vi "Routing Channel Page.vi"(8 "error in (no error)":errorcluster, 11 "Node Ptr":T6 format="%.0x") -> (0 "error out":errorcluster)   [LabVIEW 2020, in "Routing and Faulting System Explorer.lvlib"]
uses:
  Routing and Faulting System Explorer.lvlib
  <vilib>/NI VeriStand/Custom Device API/Custom Device Item Ref.ctl
  State-Value Row.ctl
  Connection Row.ctl
  State Control.ctl
  Shared/UI Common/Add Button.ctl
  Routing Channel Page Controls.ctl
  2402a215-ce2b-4427-ab28-3f6d8102afb6.vi
  Shared/Constants.vi
  Shared/UI Common/Set Control Value.vi
  <vilib>/NI VeriStand/Custom Device API/Custom Device API.lvlib
  Scripting/Routing and Faulting Scripting.lvlib
  Shared/UI Common/UI Common.lvlib
  Shared/Routing and Faulting Shared.lvlib
panel:
  in  "Configuration Tab":T1(tab)
  in  "Connections":T2[](array[typedef])
  in  "State Value":string
  in  "State Description":string
  in  "Add Connection":T3
  in  "State Name":T4
  in  "Duplicate State":bool
  in  "Remove State":bool
  in  "Add State":bool
  in  "Previous State":bool
  in  "Next State":bool
  in  "States":T5[](array[typedef])
  in  "Initial State":string(combo)
  in  "Routing Channel Name":string
  in  "SHDocVw.IWebBrowser":refnum<k7>(container)
  in  "Description":string
  # "Source"
  # "Destination"
  # "State Name"
  # "State Value"
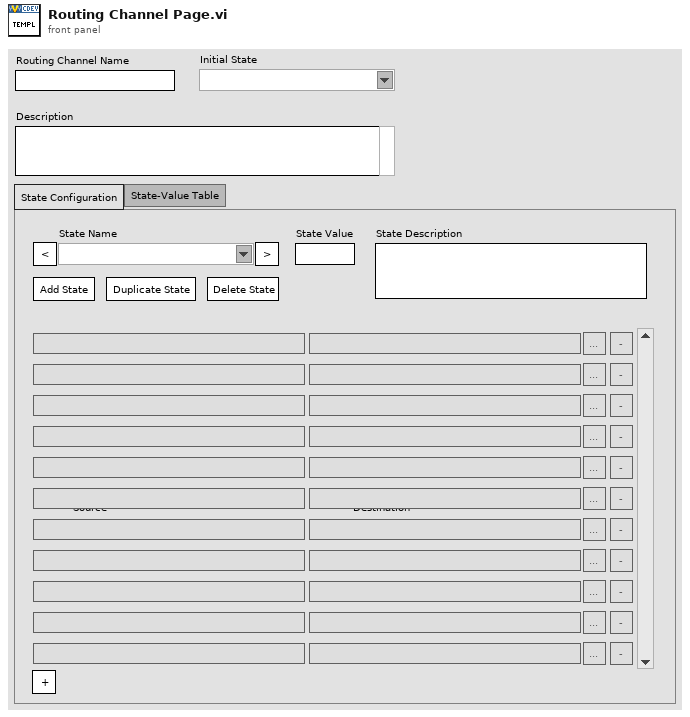
[diagram p1: front panel]
types:
  T1 = enum32{"State Configuration", "State-Value Table"}
  T2 = typedef "Routing and Faulting System Explorer.lvlib/Connection Row.ctl" = cluster{"Source":string, "Destination":string, "Edit":bool, "Remove":bool}
  T3 = typedef "UI Common.lvlib/Add Button.ctl" = bool
  T4 = typedef "Routing and Faulting System Explorer.lvlib/State Control.ctl" = string
  T5 = typedef "Routing and Faulting System Explorer.lvlib/State-Value Row.ctl" = cluster{"State":string, "State Value":string}
  T6 = typedef "Custom Device API.lvlib/Custom Device Item Ref.ctl" = u64
  T7 = typedef "Routing and Faulting System Explorer.lvlib/Routing Channel Page Controls.ctl" = cluster{"Description":refnum<vi>, "Routing Channel Name":refnum<vi>, "Initial State":refnum<vi>, "Configuration Tab":refnum<vi>, "States":refnum<vi>, "State Value":refnum<vi>, "State Name":refnum<vi>, "State Description":refnum<vi>, "Connections":refnum<vi>}
  T8 = typedef "Routing and Faulting Scripting.lvlib/Module Information.ctl" = cluster{"Module Path":string, "Product Name":string, "Possible Connections":T9[], "Configuration Revision":u32, "Validated":bool, "Missing":bool}
  T9 = typedef "Routing and Faulting Hardware API.lvlib/Possible Connections for Endpoint.ctl" = cluster{"Source":string, "Destinations":string[]}
  T10 = typedef "Routing and Faulting System Explorer.lvlib/Channel Editor State.ctl" = cluster{"Modules and Connections":T11[], "Alias Mappings UI":T12[], "Mappings by Module UI":T14[]}
  T11 = typedef "Routing and Faulting System Explorer.lvlib/Possible Connections.ctl" = cluster{" Module Path":string, "Short Module Path":string, "Product Name":string, "Possible Connections":T9[], "Missing":bool}
  T12 = typedef "Routing and Faulting Shared.lvlib/Alias Mapping.ctl" = cluster{"Alias":string, "Endpoint":T13}
  T13 = typedef "Routing and Faulting Shared.lvlib/Alias Endpoint.ctl" = cluster{"Module Path":string, "Endpoint":string}
  T14 = typedef "Routing and Faulting System Explorer.lvlib/Alias Map by Module.ctl" = cluster{"Module":string, "Alias Map":cluster{"Aliases":string[], "Endpoints":string[]}}
  T15 = typedef "Custom Device API.lvlib/Custom Device Commands.ctl" = enum16{"Default", "Item renamed", "Shutdown", "Dynamic button pressed"}
  T16 = typedef "Routing and Faulting Shared.lvlib/Connection.ctl" = cluster{"Module":string, "Source":string, "Destination":string}
  T17 = typedef "LVPoint32TypeDef.ctl" = cluster{"Horizontal":i32, "Vertical":i32}
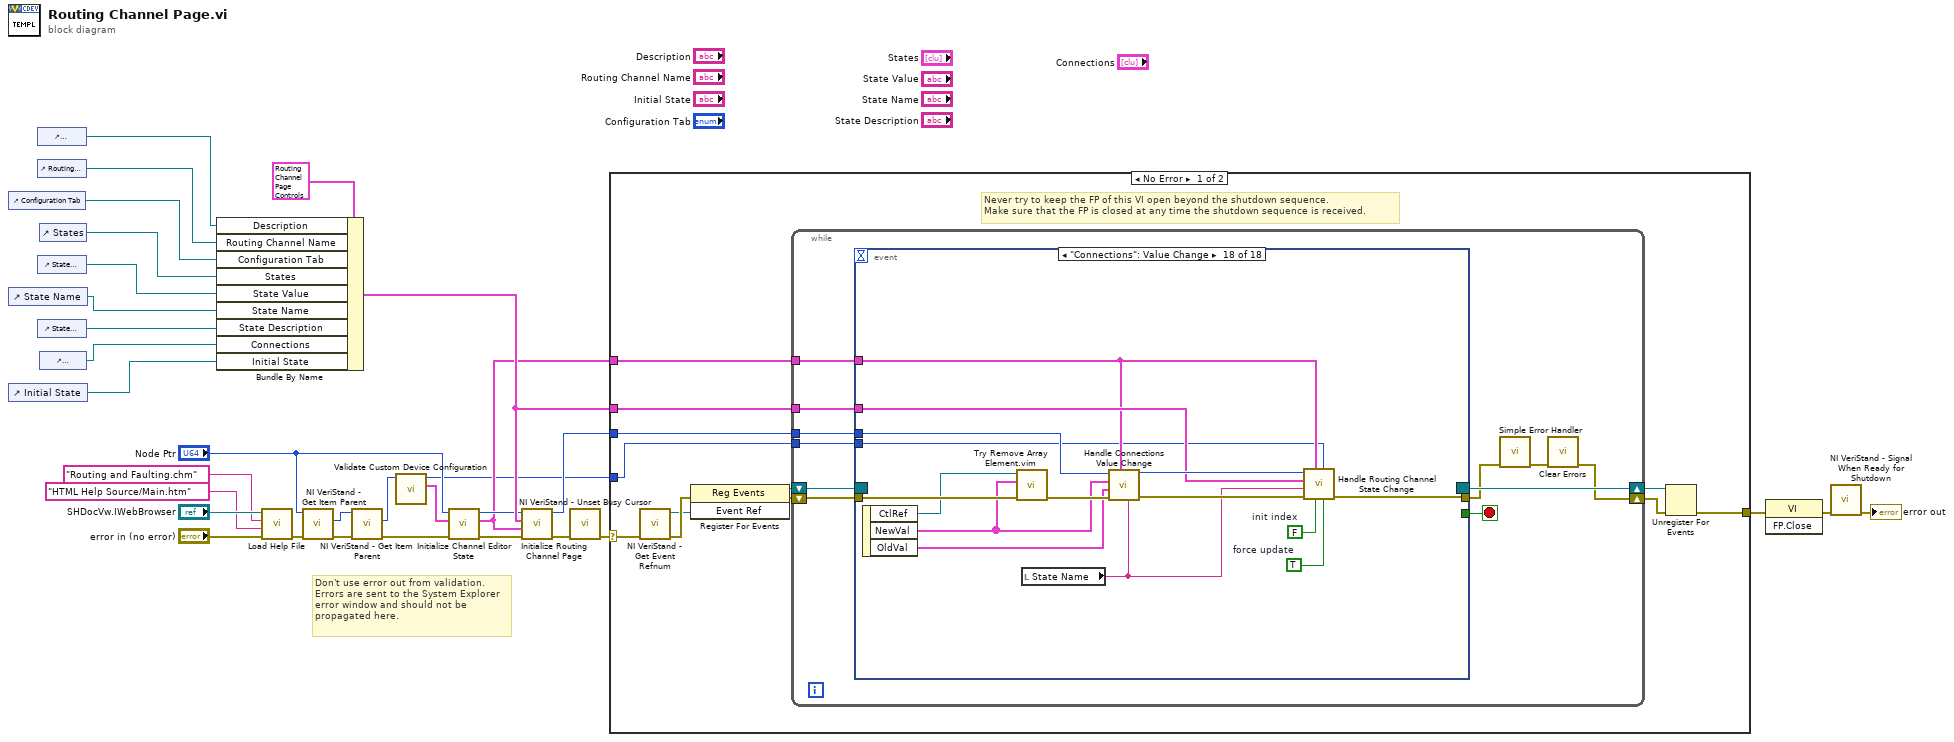
[diagram p0: block diagram]
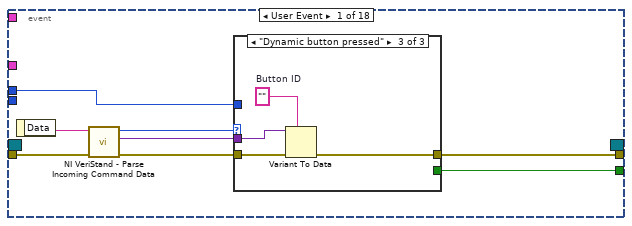
[diagram p2: hidden frame]
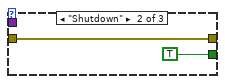
[diagram p4: hidden frame]
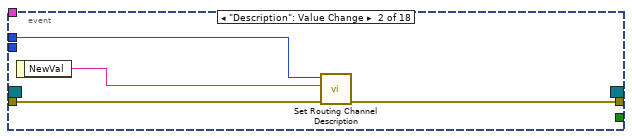
[diagram p5: hidden frame]
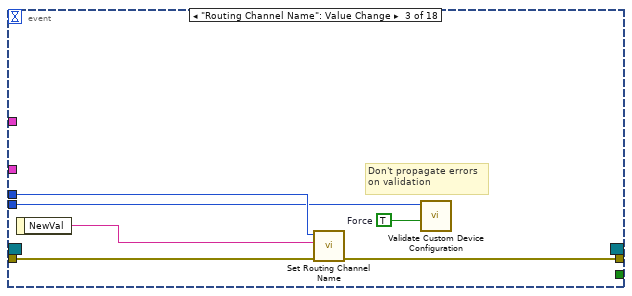
[diagram p6: hidden frame]
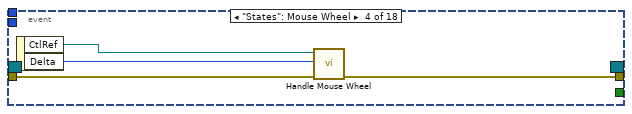
[diagram p7: hidden frame]
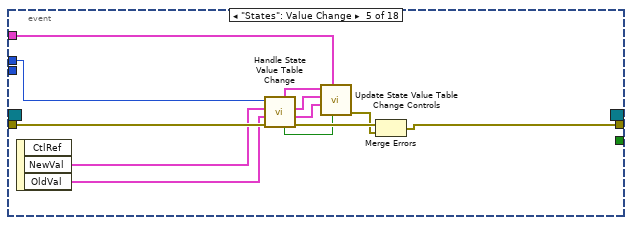
[diagram p8: hidden frame]
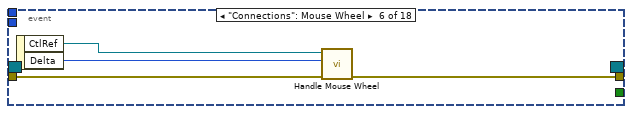
[diagram p9: hidden frame]
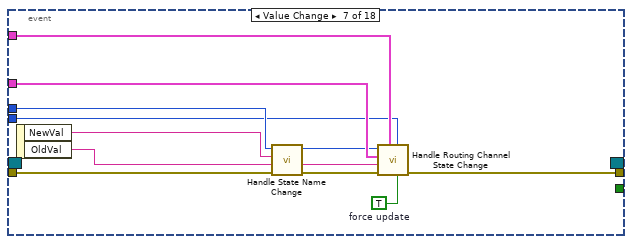
[diagram p10: hidden frame]
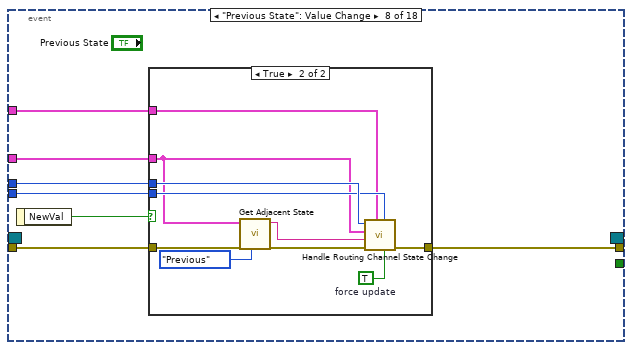
[diagram p11: hidden frame]
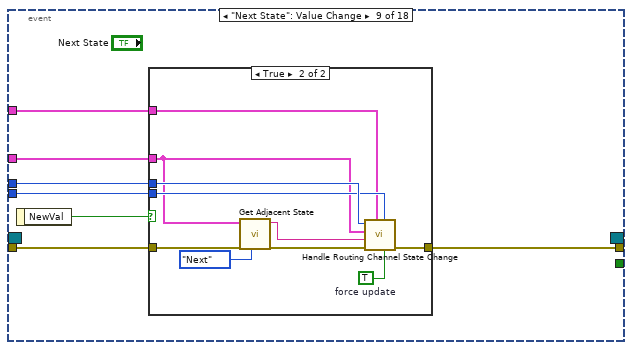
[diagram p13: hidden frame]
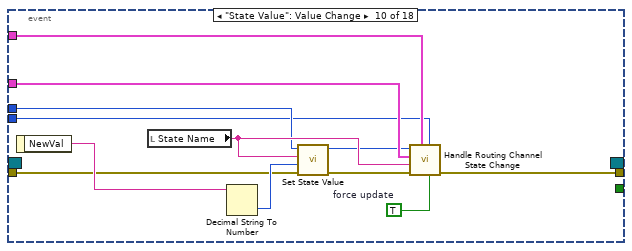
[diagram p15: hidden frame]
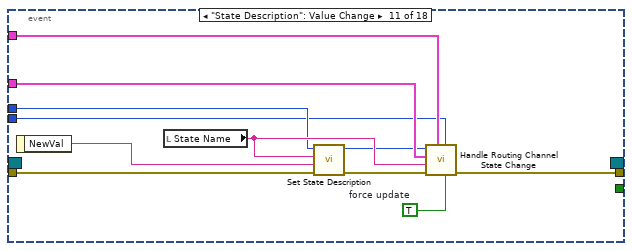
[diagram p16: hidden frame]
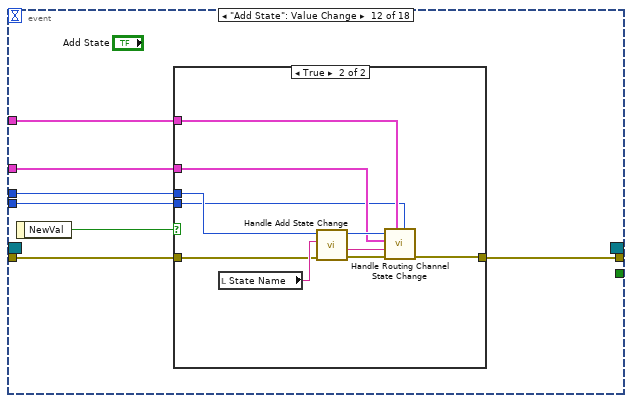
[diagram p17: hidden frame]
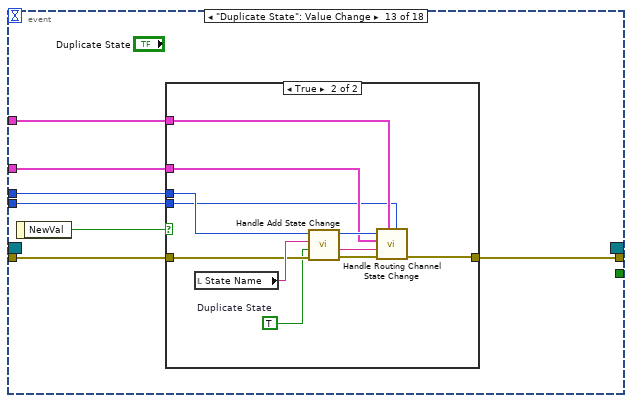
[diagram p19: hidden frame]
diagram:
  # "Don't use error out from validation.\nErrors are sent to the System Explorer\nerror window and should not be\npropagated here."
  n1 = control-ref of="Configuration Tab"() -> (w27:refnum<vi>)
  n2 = control-ref of="State Name"() -> (w18:refnum<vi>)
  n3 = control-ref of="Initial State"() -> (w14:refnum<vi>)
  n4 = control-ref of="Description"() -> (w28:refnum<vi>)
  n5 = control-ref of="Routing Channel Name"() -> (w12:refnum<vi>)
  n6 = control-ref of="State Value"() -> (w25:refnum<vi>)
  n7 = control-ref of="State Description"() -> (w13:refnum<vi>)
  n8 = control-ref of="States"() -> (w26:refnum<vi>)
  n9 = control-ref of="Connections"() -> (w19:refnum<vi>)
  n10 = Bundle By Name(cluster=T7 {"Description"=refnum, "Routing Channel Name"=refnum, "Initial State"=refnum, "Configuration Tab"=refnum, "States"=refnum, "State Value"=refnum, "State Name"=refnum, "State Description"=refnum, "Connections"=refnum} ("Routing Channel Page Controls"), "Description"=w28, "Routing Channel Name"=w12, "Configuration Tab"=w27, "States"=w26, "State Value"=w25, "State Name"=w18, "State Description"=w13, "Connections"=w19, "Initial State"=w14) -> (w15:T7)
  n11 = call "Load Help File.vi"("error in (no error)"="error in (no error)", "HTML File to Load"="HTML Help Source/Main.htm" ("HTML File"), "Main CHM File"="Routing and Faulting.chm" ("CD_CHM_FileName"), "Browser"="SHDocVw.IWebBrowser") -> ("error out"=w6:errorcluster)  [unwired: 7 in]
  n12 = call <vilib>:"NI VeriStand - Get Item Parent.vi"("error in (no error)"=w6, "Item Ref in"="Node Ptr") -> ("error out"=w7:errorcluster, "Parent Ref"=w8:T6)  [unwired: 6 in, 2 out]
  n13 = call <vilib>:"NI VeriStand - Get Item Parent.vi"("error in (no error)"=w7, "Item Ref in"=w8) -> ("error out"=w5:errorcluster, "Parent Ref"=w3:T6)  [unwired: 6 in, 2 out]
  n14 = call "Validate Custom Device Configuration.vi"("Routing and Faulting Custom Device Ref"=w3) -> ("Module Connection Information"=w4:T8[], "Routing and Faulting Custom Device Ref out"=w1:T6)  [unwired: 8 in, 1 out]
  n15 = call "Initialize Channel Editor State.vi"("error in (no error)"=w5, "Module Connection Information"=w4, "Routing Channel Ref in"="Node Ptr") -> ("error out"=w10:errorcluster, "Channel Editor State"=w9:T10, "Routing Channel Ref out"=w11:T6)  [unwired: 6 in]
  n16 = call "Initialize Routing Channel Page.vi"("error in (no error)"=w10, "Channel Editor State"=w9, "Routing Channel Page Controls"=w15, "Routing Channel Ref in"=w11) -> ("error out"=w16:errorcluster, "Routing Channel Ref out"=w17:T6)  [unwired: 6 in]
  n17 = call <vilib>:"NI VeriStand - Unset Busy Cursor.vi"("error in (no error)"=w16) -> ("error out"=w29:errorcluster)  [unwired: 10 out]
  n18 = case shown="No Error" w29 {
    selector: w29 -> [w36 w299]
    tunnel: [w41 w297] -> w32
    tunnel: w17 -> [w37 _]
    tunnel: w15 -> [w35 _]
    tunnel: w9 -> [w34 _]
    tunnel: w1 -> [w33 _]
    frame No Error {
      # "Never try to keep the FP of this VI open beyond the shutdown sequence.\nMake sure that the FP is closed at any time the shutdown sequence is received."
      n19 = call <vilib>:"NI VeriStand - Get Event Refnum.vi"("error in (no error)"=w36) -> ("error out"=w44:errorcluster, "Event Ref"=w40:refnum<user-event>)  [unwired: 9 out]
      n20 = register-events(error in=w44, w40) -> (reference out=w38:refnum<event-registration>, error out=w39:errorcluster)  [unwired: 1 in]
      n21 = while {
        tunnel: w37 -> [w51]
        shift-right: [w48] -> w42
        shift-left: w39 -> [w54]
        shift-right: [w55] -> w43
        shift-left: w38 -> [w53]
        tunnel: w35 -> [w47]
        tunnel: w34 -> [w46]
        tunnel: w33 -> [w45]
        stop <- w52 stop-if-true
        n22 = event shown="[17] \"Connections\": Value Change" {
          selector: w53 -> [_ _ _ _ _ _ _ _ _ _ _ _ _ _ _ _ _ _]
          dyn-events: [_ _ _ _ _ _ _ _ _ _ _ _ _ _ _ _ _ _] -> w55
          timeout: _ -> [_ _ _ _ _ _ _ _ _ _ _ _ _ _ _ _ _ _]
          tunnel: w54 -> [w63 w73 w79 w83 w96 w99 w110 w119 w137 w156 w169 w177 w195 w213 w235 w243 _ w296]
          tunnel: [w59 _ _ _ _ _ _ _ _ _ _ _ _ _ _ _ _ _] -> w52
          tunnel: [w58 w72 w75 w84 w86 w100 w112 w118 w136 w160 w171 w176 w194 w212 w234 w241 _ w289] -> w50
          tunnel: w51 -> [w57 w74 w80 _ w92 _ w107 w115 w133 w153 w166 w178 w196 w215 w231 w245 _ w294]
          tunnel: w47 -> [_ _ _ _ w90 _ w111 w116 w134 w159 w170 w174 w192 w214 w236 w242 _ w287]
          tunnel: w46 -> [_ _ _ _ _ _ w102 w114 w132 w150 w162 w173 w191 w210 w228 w238 w260 w283]
          tunnel: w45 -> [_ _ w77 _ _ _ w101 w113 w131 w149 w161 w172 w190 w209 w227 w237 _ w282]
          event User Event {
            n23 = event-data() -> ("Data"=w62:string)  [unwired: 1 out]
            n24 = call <vilib>:"NI VeriStand - Parse Incoming Command Data.vi"("error in (no error)"=w63, "Incoming data"=w62) -> ("error out"=w61:errorcluster, "Outgoing data"=w56:variant, "Action"=w60:T15)  [unwired: 7 out]
            n25 = case shown="\"Dynamic button pressed\"" w60 {
              tunnel: w61 -> [w64 w65 w70]
              tunnel: [_ TRUE _] -> w59
              tunnel: [w64 w65 w67] -> w58
              tunnel: w57 -> [_ _ _]
              tunnel: w56 -> [_ _ w69]
              frame "Default", Default {
              }
              frame "Shutdown" {
              }
              frame "Dynamic button pressed" {
                w68 = ""  # Button ID
                n26 = Variant To Data(error in=w70, type=w68, Variant=w69) -> (error out=w67:errorcluster)  [unwired: 1 out]
              }
            }
          }
          event "Description": Value Change {
            n27 = event-data() -> ("NewVal"=w71:string)  [unwired: 1 out]
            n28 = call "Set Routing Channel Description.vi"("error in"=w73, "description"=w71, "routing channel in"=w74) -> ("error out"=w72:errorcluster)  [unwired: 7 in, 1 out]
          }
          event "Routing Channel Name": Value Change {
            w76 = TRUE  # Force
            # "Don't propagate errors\non validation"
            n29 = event-data() -> ("NewVal"=w78:string)  [unwired: 1 out]
            n30 = call "Set Routing Channel Name.vi"("error in"=w79, "routing channel name"=w78, "routing channel in"=w80) -> ("error out"=w75:errorcluster)  [unwired: 7 in, 1 out]
            n31 = call "Validate Custom Device Configuration.vi"("Force Validation (F)"=w76, "Routing and Faulting Custom Device Ref"=w77) -> ()  [unwired: 7 in, 3 out]
          }
          event "States": Mouse Wheel {
            n32 = event-data() -> ("CtlRef"=w82:refnum<vi>, "Delta"=w81:i32)  [unwired: 1 out]
            n33 = call "Handle Mouse Wheel.vi"("error in (no error)"=w83, "delta"=w81, "Array Refnum"=w82) -> ("error out"=w84:errorcluster)  [unwired: 7 in, 1 out]
          }
          event "States": Value Change {
            n34 = event-data() -> ("NewVal"=w94:T5[], "OldVal"=w93:T5[])  [unwired: 2 out]
            n35 = call "Handle State Value Table Change.vi"("error in (no error)"=w96, "OldVal"=w93, "NewVal"=w94, "routing channel in"=w92) -> ("error out"=w95:errorcluster, "old modified state and value"=w88:T5, "new modified state and value"=w89:T5, "update controls"=w87:bool, "coerced newval"=w91:T5[])  [unwired: 2 in, 1 out]
            n36 = call "Update State Value Table Change Controls.vi"("update all controls?"=w87, "Routing Channel Page Controls"=w90, "old modified state and value"=w88, "new modified state and value"=w89, "all states and values"=w91) -> ("error out"=w85:errorcluster)  [unwired: 6 in]
            n37 = Merge Errors(w95, w85) -> (w86:errorcluster)
          }
          event "Connections": Mouse Wheel {
            n38 = event-data() -> ("CtlRef"=w97:refnum<vi>, "Delta"=w98:i32)  [unwired: 1 out]
            n39 = call "Handle Mouse Wheel.vi"("error in (no error)"=w99, "delta"=w98, "Array Refnum"=w97) -> ("error out"=w100:errorcluster)  [unwired: 7 in, 1 out]
          }
          event Value Change {
            w103 = TRUE  # force update
            n40 = event-data() -> ("NewVal"=w109:T4, "OldVal"=w108:T4)  [unwired: 1 out]
            n41 = call "Handle State Name Change.vi"("error in (no error)"=w110, "Old State Name"=w108, "New State Name"=w109, "Routing Channel Ref in"=w107) -> ("error out"=w106:errorcluster, "State to Display"=w104:string, "Routing Channel Ref out"=w105:T6)  [unwired: 5 in]
            n42 = call "Handle Routing Channel State Change.vi"("force update"=w103, "Routing and Faulting Custom Device Ref"=w101, "Channel Editor State"=w102, "error in (no error)"=w106, "State"=w104, "Routing Channel Page Controls"=w111, "Routing Channel Ref in"=w105) -> ("error out"=w112:errorcluster)  [unwired: 3 in, 1 out]
          }
          event "Previous State": Value Change {
            n43 = event-data() -> ("NewVal"=w117:bool)  [unwired: 1 out]
            n44 = case shown="True" w117 {
              tunnel: w119 -> [w120 w123]
              tunnel: [w120 w129] -> w118
              tunnel: w116 -> [_ w125]
              tunnel: w115 -> [_ w128]
              tunnel: w114 -> [_ w126]
              tunnel: w113 -> [_ w127]
              frame False {
              }
              frame True {
                w130 = TRUE  # force update
                n45 = call "Get Adjacent State.vi"("Direction"=enum16{"Previous", "Next"}."Previous", "error in (no error)"=w123, "Routing Channel Page Controls"=w125) -> ("error out"=w124:errorcluster, "state name"=w122:string)  [unwired: 7 in]
                n46 = call "Handle Routing Channel State Change.vi"("force update"=w130, "Routing and Faulting Custom Device Ref"=w127, "Channel Editor State"=w126, "error in (no error)"=w124, "State"=w122, "Routing Channel Page Controls"=w125, "Routing Channel Ref in"=w128) -> ("error out"=w129:errorcluster)  [unwired: 3 in, 1 out]
              }
            }
          }
          event "Next State": Value Change {
            n47 = event-data() -> ("NewVal"=w135:bool)  [unwired: 1 out]
            n48 = case shown="True" w135 {
              tunnel: w137 -> [w138 w141]
              tunnel: [w138 w147] -> w136
              tunnel: w134 -> [_ w143]
              tunnel: w133 -> [_ w146]
              tunnel: w132 -> [_ w144]
              tunnel: w131 -> [_ w145]
              frame False {
              }
              frame True {
                w148 = TRUE  # force update
                n49 = call "Get Adjacent State.vi"("Direction"=enum16{"Previous", "Next"}."Next", "error in (no error)"=w141, "Routing Channel Page Controls"=w143) -> ("error out"=w142:errorcluster, "state name"=w140:string)  [unwired: 7 in]
                n50 = call "Handle Routing Channel State Change.vi"("force update"=w148, "Routing and Faulting Custom Device Ref"=w145, "Channel Editor State"=w144, "error in (no error)"=w142, "State"=w140, "Routing Channel Page Controls"=w143, "Routing Channel Ref in"=w146) -> ("error out"=w147:errorcluster)  [unwired: 3 in, 1 out]
              }
            }
          }
          event "State Value": Value Change {
            w151 = TRUE  # force update
            n51 = event-data() -> ("NewVal"=w157:string)  [unwired: 1 out]
            n52 = local read "State Name"() -> (w154:T4)
            n53 = Decimal String To Number(string=w157) -> (number=w158:i32)  [unwired: 2 in, 1 out]
            n54 = call "Set State Value.vi"("error in"=w156, "value"=w158, "state"=w154, "routing channel in"=w153) -> ("error out"=w155:errorcluster, "routing channel out"=w152:T6)  [unwired: 6 in]
            n55 = call "Handle Routing Channel State Change.vi"("force update"=w151, "Routing and Faulting Custom Device Ref"=w149, "Channel Editor State"=w150, "error in (no error)"=w155, "State"=w154, "Routing Channel Page Controls"=w159, "Routing Channel Ref in"=w152) -> ("error out"=w160:errorcluster)  [unwired: 3 in, 1 out]
          }
          event "State Description": Value Change {
            w164 = TRUE  # force update
            n56 = event-data() -> ("NewVal"=w163:string)  [unwired: 1 out]
            n57 = local read "State Name"() -> (w167:T4)
            n58 = call "Set State Description.vi"("error in"=w169, "descriptions"=w163, "state"=w167, "routing channel in"=w166) -> ("error out"=w168:errorcluster, "routing channel out"=w165:T6)  [unwired: 6 in]
            n59 = call "Handle Routing Channel State Change.vi"("force update"=w164, "Routing and Faulting Custom Device Ref"=w161, "Channel Editor State"=w162, "error in (no error)"=w168, "State"=w167, "Routing Channel Page Controls"=w170, "Routing Channel Ref in"=w165) -> ("error out"=w171:errorcluster)  [unwired: 3 in, 1 out]
          }
          event "Add State": Value Change {
            n60 = event-data() -> ("NewVal"=w175:bool)  [unwired: 1 out]
            n61 = case shown="True" w175 {
              tunnel: w178 -> [_ w189]
              tunnel: w174 -> [_ w185]
              tunnel: w177 -> [w179 w183]
              tunnel: [w179 w184] -> w176
              tunnel: w173 -> [_ w181]
              tunnel: w172 -> [_ w180]
              frame False {
              }
              frame True {
                n62 = local read "State Name"() -> (w188:T4)
                n63 = call "Handle Add State Change.vi"("error in (no error)"=w183, "State"=w188, "Routing Channel Ref in"=w189) -> ("error out"=w186:errorcluster, "New State Added"=w182:string, "Routing Channel Ref out"=w187:T6)  [unwired: 6 in]
                n64 = call "Handle Routing Channel State Change.vi"("Routing and Faulting Custom Device Ref"=w180, "Channel Editor State"=w181, "error in (no error)"=w186, "State"=w182, "Routing Channel Page Controls"=w185, "Routing Channel Ref in"=w187) -> ("error out"=w184:errorcluster)  [unwired: 4 in, 1 out]
              }
            }
          }
          event "Duplicate State": Value Change {
            n65 = event-data() -> ("NewVal"=w193:bool)  [unwired: 1 out]
            n66 = case shown="True" w193 {
              tunnel: w196 -> [_ w208]
              tunnel: w192 -> [_ w204]
              tunnel: w195 -> [w197 w202]
              tunnel: [w197 w203] -> w194
              tunnel: w191 -> [_ w199]
              tunnel: w190 -> [_ w198]
              frame False {
              }
              frame True {
                w200 = TRUE  # Duplicate State
                n67 = local read "State Name"() -> (w207:T4)
                n68 = call "Handle Add State Change.vi"("error in (no error)"=w202, "Duplicate State"=w200, "State"=w207, "Routing Channel Ref in"=w208) -> ("error out"=w205:errorcluster, "New State Added"=w201:string, "Routing Channel Ref out"=w206:T6)  [unwired: 5 in]
                n69 = call "Handle Routing Channel State Change.vi"("Routing and Faulting Custom Device Ref"=w198, "Channel Editor State"=w199, "error in (no error)"=w205, "State"=w201, "Routing Channel Page Controls"=w204, "Routing Channel Ref in"=w206) -> ("error out"=w203:errorcluster)  [unwired: 4 in, 1 out]
              }
            }
          }
          event "Remove State": Value Change {
            n70 = event-data() -> ("NewVal"=w211:bool)  [unwired: 1 out]
            n71 = case shown="True" w211 {
              tunnel: w215 -> [_ w226]
              tunnel: w214 -> [_ w222]
              tunnel: w213 -> [w216 w220]
              tunnel: [w216 w221] -> w212
              tunnel: w210 -> [_ w218]
              tunnel: w209 -> [_ w217]
              frame False {
              }
              frame True {
                n72 = local read "State Name"() -> (w225:T4)
                n73 = call "Handle Remove State Change.vi"("error in (no error)"=w220, "State"=w225, "Routing Channel Ref in"=w226) -> ("error out"=w223:errorcluster, "State to Display"=w219:string, "Routing Channel Ref out"=w224:T6)  [unwired: 6 in]
                n74 = call "Handle Routing Channel State Change.vi"("Routing and Faulting Custom Device Ref"=w217, "Channel Editor State"=w218, "error in (no error)"=w223, "State"=w219, "Routing Channel Page Controls"=w222, "Routing Channel Ref in"=w224) -> ("error out"=w221:errorcluster)  [unwired: 4 in, 1 out]
              }
            }
          }
          event "Initial State": Value Change {
            n75 = event-data() -> ("NewVal"=w229:string)  [unwired: 1 out]
            n76 = call "Set Routing Channel Initial State.vi"("error in"=w235, "state"=w229, "routing channel in"=w231) -> ("error out"=w232:errorcluster, "routing channel out"=w230:T6)  [unwired: 7 in]
            n77 = local read "State Name"() -> (w233:T4)
            n78 = call "Handle Routing Channel State Change.vi"("Routing and Faulting Custom Device Ref"=w227, "Channel Editor State"=w228, "error in (no error)"=w232, "State"=w233, "Routing Channel Page Controls"=w236, "Routing Channel Ref in"=w230) -> ("error out"=w234:errorcluster)  [unwired: 4 in, 1 out]
          }
          event Value Change {
            n79 = event-data() -> ()  [unwired: 2 out]
            n80 = call "Configure Connection Dialog.vi"("error in (no error)"=w243, "Channel Editor State"=w238) -> ("error out"=w244:errorcluster, "Connection (R,S,D)"=w239:T16, "Canceled?"=w240:bool)  [unwired: 7 in]
            n81 = case shown="False" w240 {
              tunnel: w245 -> [w253 _]
              tunnel: w239 -> [w249 _]
              tunnel: w244 -> [w250 w257]
              tunnel: w242 -> [w255 _]
              tunnel: [w252 w257] -> w241
              tunnel: w238 -> [w247 _]
              tunnel: w237 -> [w246 _]
              frame False {
                w248 = FALSE  # init index
                n82 = local read "State Name"() -> (w251:T4)
                n83 = call "Add Connection to State.vi"("error in"=w250, "connection"=w249, "state"=w251, "routing channel in"=w253) -> ("error out"=w256:errorcluster, "routing channel out"=w254:T6)  [unwired: 6 in]
                n84 = call "Handle Routing Channel State Change.vi"("Routing and Faulting Custom Device Ref"=w246, "init index"=w248, "Channel Editor State"=w247, "error in (no error)"=w256, "State"=w251, "Routing Channel Page Controls"=w255, "Routing Channel Ref in"=w254) -> ("error out"=w252:errorcluster)  [unwired: 3 in, 1 out]
              }
              frame True {
              }
            }
          }
          event "Connections": Mouse Move {
            n85 = event-data() -> ("CtlRef"=w261:refnum<vi>, "Coords"=w262:T17)  [unwired: 1 out]
            n86 = global read "Constants.vi" "Tip-Strip Update Period"() -> (w259:dbl)
            n87 = call "Elapsed Time"("Time Target (s)"=w259) -> ("Time has Elapsed"=w258:bool)  [unwired: 11 in, 7 out]
            n88 = case shown="True" w258 {
              tunnel: w262 -> [_ w269]
              tunnel: w261 -> [_ w268]
              tunnel: w260 -> [_ w267]
              frame False {
                # "Handle Mouse Move only every 10ms"
              }
              frame True {
                n89 = call "Get Mouse Location (Connections).vi"("Event Coord"=w269, "Connections Reference"=w268) -> ("in data range"=w263:bool, "Element Reference"=w264:refnum<vi>, "Type"=w266:enum16{"Source", "Destination", "Neither"}, "Array Index"=w265:i32)  [unwired: 6 in]
                n90 = case shown="\"Source\", \"Destination\"" w266 {
                  selector: w266 -> [_ w273]
                  tunnel: w267 -> [_ w274]
                  tunnel: w265 -> [_ w275]
                  tunnel: w264 -> [_ w271]
                  tunnel: w263 -> [_ w270]
                  frame Default {
                  }
                  frame "Source", "Destination" {
                    n91 = case shown="True" w270 {
                      tunnel: w275 -> [_ w280]
                      tunnel: w274 -> [_ w278]
                      tunnel: w273 -> [_ w277]
                      tunnel: [_ w276] -> w272
                      frame False {
                      }
                      frame True {
                        n92 = local read "Connections"() -> (w281:T2[])
                        n93 = Index Array(array=w281, index=w280) -> (element=w279:T2)
                        n94 = call "Get Alias-Free Connection Endpoint.vi"("type"=w277, "Connection row"=w279, "Channel Editor State"=w278) -> ("Endpoint (Model) String"=w276:string)  [unwired: 8 in]
                      }
                    }
                    n95 = property class="Ctl"(reference=w271, "TipStrip"=w272) -> ()  [unwired: 1 in, 2 out]
                  }
                }
              }
            }
          }
          event "Connections": Value Change {
            w284 = TRUE  # force update
            w291 = FALSE  # init index
            n96 = event-data() -> ("CtlRef"=w286:refnum<vi>, "NewVal"=w293:T2[], "OldVal"=w292:T2[])  [unwired: 1 out]
            n97 = call "Try Remove Array Element.vim"("error in (no error)"=w296, "Array"=w293, "Ctl Refnum"=w286) -> ("error out"=w295:errorcluster)  [unwired: 6 in, 2 out]
            n98 = local read "State Name"() -> (w285:T4)
            n99 = call "Handle Connections Value Change.vi"("State"=w285, "Channel Editor State"=w283, "error in (no error)"=w295, "OldVal"=w292, "NewVal"=w293, "Routing Channel Ref in"=w294) -> ("error out"=w290:errorcluster, "Routing Channel Ref out"=w288:T6)  [unwired: 4 in]
            n100 = call "Handle Routing Channel State Change.vi"("force update"=w284, "Routing and Faulting Custom Device Ref"=w282, "init index"=w291, "Channel Editor State"=w283, "error in (no error)"=w290, "State"=w285, "Routing Channel Page Controls"=w287, "Routing Channel Ref in"=w288) -> ("error out"=w289:errorcluster)  [unwired: 2 in, 1 out]
          }
        }
        n101 = call <vilib>:"Simple Error Handler.vi"("error in (no error)"=w50) -> ("error out"=w49:errorcluster)  [unwired: 1 in, 7 out]
        n102 = call <vilib>:"Clear Errors.vi"("error in (no error)"=w49) -> ("error out"=w48:errorcluster)  [unwired: 1 in, 5 out]
      }
      n103 = Unregister For Events(event registration refnum=w43, error in=w42) -> (error out=w41:errorcluster)
    }
    frame Error {
      n104 = call <vilib>:"Simple Error Handler.vi"("error in (no error)"=w299) -> ("error out"=w298:errorcluster)  [unwired: 1 in, 7 out]
      n105 = call <vilib>:"Clear Errors.vi"("error in (no error)"=w298) -> ("error out"=w297:errorcluster)  [unwired: 1 in, 5 out]
    }
  }
  n106 = invoke class="VI" method="FP.Close"(error in=w32) -> (error out=w31:errorcluster)  [unwired: 2 in, 2 out]
  n107 = call <vilib>:"NI VeriStand - Signal When Ready for Shutdown.vi"("error in (no error)"=w31) -> ("error out"=→"error out":errorcluster)  [unwired: 10 out]
